vi "Monitor Pressure & Flow.vi"() -> ()   [LabVIEW 2011, in "MGC647C.lvlib"]
doc: "This sample VI illustrates the usage of the driver to monitor pressure and flow values as well as channel status."
uses:
  <instrlib>/MGC647C/MGC647C.lvlib
panel:
  in  "#Channels":i32=4
  in  "Interval":dbl[unit]
  in  "Stop":bool
  out "Trend Chart":T1(graph)
  out "Flow Channels":T2(array[cluster])
  out "Actual Pressure":dbl[unit]
  in  "Serial Configuration":T3={"Baud Rate"=9600, "Parity"=0, "Data Bits"=8, "Stop Bits"=10, "Flow Control"=0} {"Flow Control" items=["None", "XON/XOFF", "RTS/CTS", "XON/XOFF & RTS/CTS", "DTR/DSR", "XON/XOFF & DTR/DSR"]; "Stop Bits" items=["1.0"=10, "1.5"=15, "2.0"=20]; "Data Bits" items=["7"=7, "8"=8]; "Parity" items=["None", "Odd", "Even", "Mark", "Space"]; "Baud Rate" items=["300"=300, "600"=600, "1200"=1200, "2400"=2400, "4800"=4800, "9600"=9600, "19200"=19200]}
  in  "Set Defaults? (F)":bool
  in  "Reset (True)":bool
  in  "ID Query (True)":bool=TRUE
  in  "VISA resource name":refnum<visa-resource-name>
  # "(C) Copyright 2012 GSI Helmholtzzentrum für Schwerionenforschung GmbH.  ALL RIGHTS RESERVED."
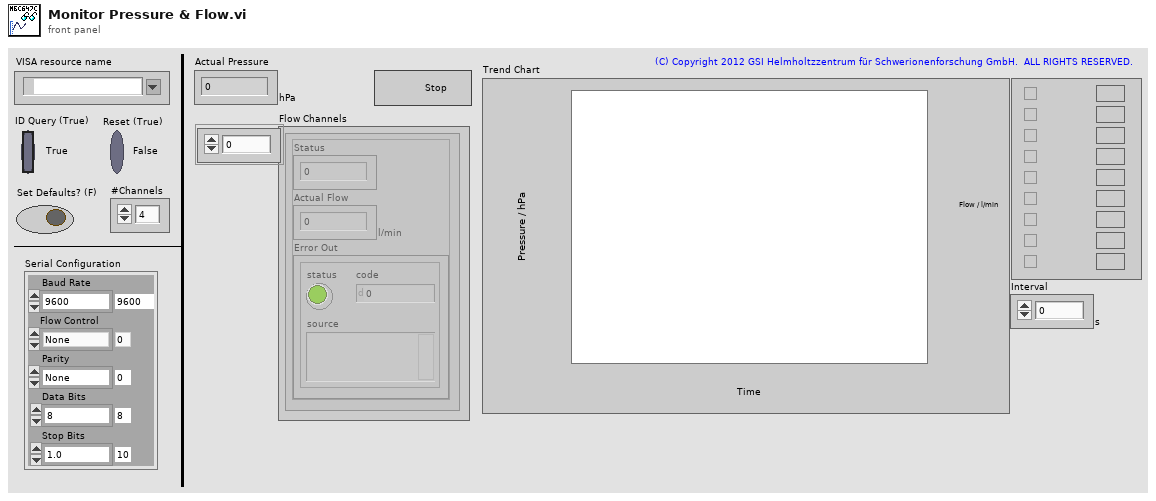
[diagram p1: front panel]
types:
  T1 = cluster{"[0]":dbl, "[1]":dbl, "[2]":dbl, "[3]":dbl, "[4]":dbl, "[5]":dbl, "[6]":dbl, "[7]":dbl, "[8]":dbl}
  T2 = cluster{"Status":u16, "Actual Flow":dbl[unit], "Error Out":errorcluster}[]
  T3 = cluster{"Baud Rate":u32, "Parity":u16, "Data Bits":u16, "Stop Bits":u16, "Flow Control":u16}
  T4 = cluster{"Status":u16, "Flow":dbl[unit], "Error Out":errorcluster}
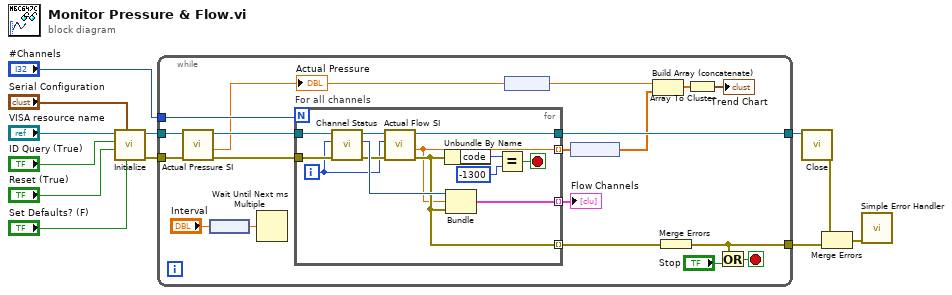
[diagram p0: block diagram]
diagram:
  n1 = call <instrlib>:"Initialize.vi"("Set Defaults? (F)"="Set Defaults? (F)", "Serial Configuration"="Serial Configuration", "Reset (True)"="Reset (True)", "ID Query (True)"="ID Query (True)", "VISA resource name"="VISA resource name") -> ("error out"=w6:errorcluster, "VISA resource name out"=w7:refnum<visa-resource-name>)  [unwired: 5 in]
  n2 = while {
    tunnel: w7 -> [w21]
    tunnel: w6 -> [w20]
    tunnel: [w22] -> w2
    tunnel: [w29] -> w5
    tunnel: "#Channels" -> [w26]
    stop <- w25 stop-if-true
    n3 = call <instrlib>:"Actual Pressure SI.vi"("Error In"=w20, "VISA resource name"=w21) -> ("Error Out"=w19:errorcluster, "Pressure"=w17:dbl[unit], "dup VISA resource name"=w18:refnum<visa-resource-name>)  [unwired: 7 in]
    "Actual Pressure" <- w17
    n4 = node("Interval") -> (w27:dbl)
    n5 = Wait Until Next ms Multiple(millisecond multiple=w27) -> ()  [unwired: 1 out]
    n6 = for "For all channels" {
      N: w26 -> [_]
      tunnel: w18 -> [w44]
      tunnel: w19 -> [w43]
      tunnel: [w38] -> w13 mode=indexing
      tunnel: [w33] -> w15 mode=indexing
      tunnel: [w34] -> w31 mode=indexing
      tunnel: [w35] -> w29
      i -> [w32]
      stop <- w40 stop-if-true
      n7 = call <instrlib>:"Channel Status.vi"("Error In"=w43, "Channel (-1:Main)"=w32, "VISA resource name"=w44) -> ("Error Out"=w36:errorcluster, "Status"=w39:u16, "dup VISA resource name"=w37:refnum<visa-resource-name>)  [unwired: 5 in, 1 out]
      n8 = call <instrlib>:"Actual Flow SI.vi"("Error In"=w36, "Channel (0)"=w32, "VISA resource name"=w37) -> ("Error Out"=w34:errorcluster, "Flow"=w33:dbl[unit], "dup VISA resource name"=w35:refnum<visa-resource-name>)  [unwired: 6 in]
      n9 = Unbundle By Name(w34) -> ("code"=w42:i32)
      n10 = Bundle("Status"=w39, "Flow"=w33, "Error Out"=w34) -> (w38:T4)  [unwired: 1 in]
      n11 = Equal?(x=w42, y=-1300) -> (x = y?=w40:bool)
    }
    "Flow Channels" <- w13
    n12 = node(w17) -> (w16:dbl)
    n13 = node(w15) -> (w14:dbl[])
    n14 = Build Array (concatenate)(w16, w14) -> (w24:dbl[])
    n15 = Merge Errors(w31) -> (w22:errorcluster)
    n16 = Array To Cluster(array=w24) -> (cluster=→"Trend Chart":T1)
    n17 = Or(x=w22, y="Stop") -> (x .or. y?=w25:bool)
  }
  n18 = call <instrlib>:"Close.vi"("VISA resource name"=w5) -> ("error out"=w4:errorcluster)  [unwired: 10 in]
  n19 = Merge Errors(w4, w2) -> (w3:errorcluster)
  n20 = call <vilib>:"Simple Error Handler.vi"("error in (no error)"=w3) -> ()  [unwired: 4 in, 5 out]
